vi "Open Config Data (compatibility).vi"(8 "error in (no error)":errorcluster, 10 "create file if necessary (T)":bool=TRUE, 11 "configuration file path":path) -> (0 "error out":errorcluster, 2 "file created?":bool, 3 "refnum":T1)   [LabVIEW 2017, in "NI_LVConfig.lvlib"]
doc: "The Open Config Data VI was rewritten with one new output in LabVIEW 2009 and later. Replace the Open Config Data (compatibility) VI with an Open Config Data VI from the Functions palette to use the new functionality."
uses:
  <vilib>/Utility/config.llb/NI_LVConfig.lvlib
  <vilib>/Utility/config.llb/Config Data RefNum.ctl
  <vilib>/Utility/config.llb/Config Data.ctl
  <vilib>/Utility/config.llb/Section.ctl
  <vilib>/Utility/config.llb/8.6CompatibleGlobalVar.vi
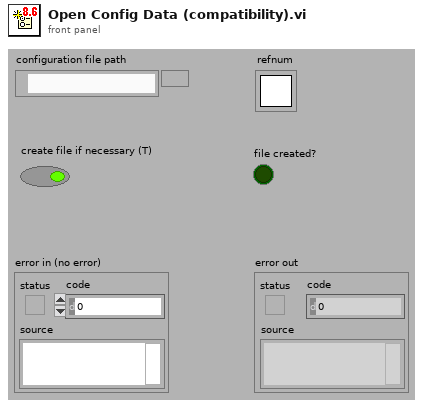
[diagram p1: front panel]
types:
  T1 = typedef "NI_LVConfig.lvlib/Config Data RefNum.ctl" = refnum<k1>
  T2 = typedef "NI_LVConfig.lvlib/Config Data.ctl" = cluster{"sections":T3[], "path":path, "dirty":bool}
  T3 = typedef "NI_LVConfig.lvlib/Section.ctl" = cluster{"name":string, "comment":string, "kvc":string[][]}
  T4 = typedef "NI_LVConfig.lvlib/Config Queue.ctl" = refnum<queue>
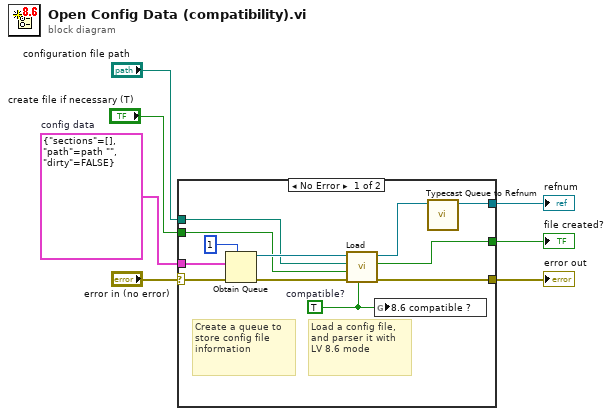
[diagram p0: block diagram]
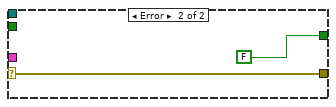
[diagram p2: hidden frame]
diagram:
  w1 = T2 {"sections"=[], "path"=path "", "dirty"=FALSE}  # config data
  n1 = case shown="No Error" "error in (no error)" {
    selector: "error in (no error)" -> [w18 w21]
    tunnel: "configuration file path" -> [w14 _]
    tunnel: "create file if necessary (T)" -> [w13 _]
    tunnel: [w10 FALSE ("file created?")] -> w3
    tunnel: [w11 w21] -> w4
    tunnel: w1 -> [w17 _]
    tunnel: [w16 _] -> w2
    frame No Error {
      w8 = TRUE  # compatible?
      # "Load a config file, and parser it with LV 8.6 mode"
      # "Create a queue to store config file information"
      n2 = Obtain Queue(max queue size (-1, unlimited)=1, element data type=w17, error in (no error)=w18) -> (queue out=w15:refnum<queue>, error out=w12:errorcluster)  [unwired: 2 in, 1 out]
      n3 = call <vilib>:"Load.vi"("compatible?"=w8, "error in (no error)"=w12, "create file if necessary? (T)"=w13, "configuration file path"=w14, "queue in"=w15) -> ("error out"=w11:errorcluster, "file created?"=w10:bool, "queue out"=w9:T4)  [unwired: 4 in]
      n4 = global write "8.6CompatibleGlobalVar.vi" "8.6 compatible ?"(w8) -> ()
      n5 = call <vilib>:"Typecast Queue to Refnum.vi"("queue in"=w9) -> ("refnum out"=w16:T1)  [unwired: 10 in]
    }
    frame Error {
    }
  }
  "error out" <- w4
  "file created?" <- w3
  "refnum" <- w2
